vi "ReadFileONLY.vi"(8 "error in (no error)":errorcluster, 10 "file path (dialog if empty)":path) -> (0 "error out":errorcluster, 1 "Waveform Graph":waveform(dbl)[](graph), 2 "number of waveforms":i32, 3 "Array":string[](array[string]), 4 "saturated":bool[](array[boolean]), 5 "dX/dt 2":dbl[](graph))   [LabVIEW 2013]
uses:
  <instrlib>/niHWS/nihws.llb/niHWS Open File Permissions ID.ctl
  <instrlib>/niHWS/nihws.llb/niHWS Read Analog WDT.vi
panel:
  out "Array 2":dbl[](array[numeric]) format="%#_6p"
  in  "index (row)":i32
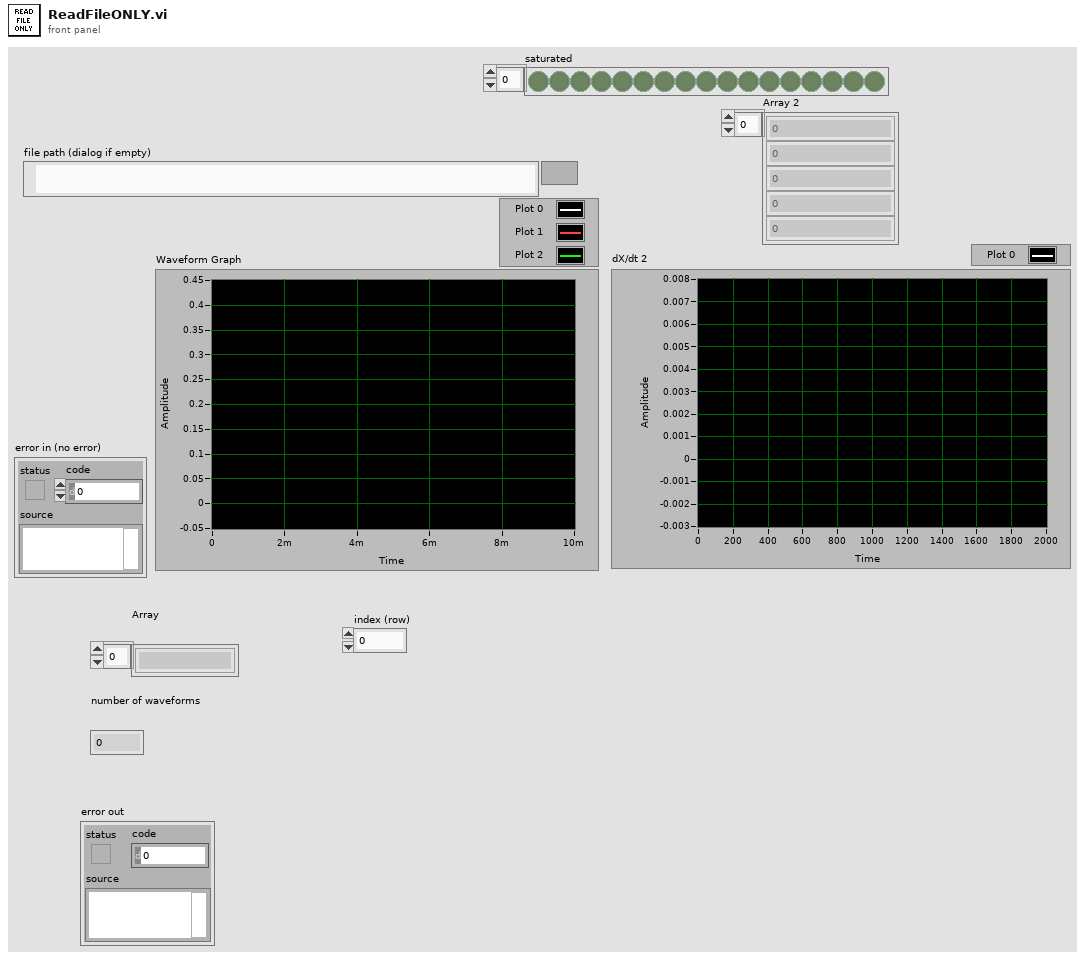
[diagram p1: front panel]
types:
  T1 = typedef "niHWS Open File Permissions ID.ctl" = enum32{"Read Only", "Read/Write Existing", "Read/Write/Create New", "Read/Write/Create New Always"}
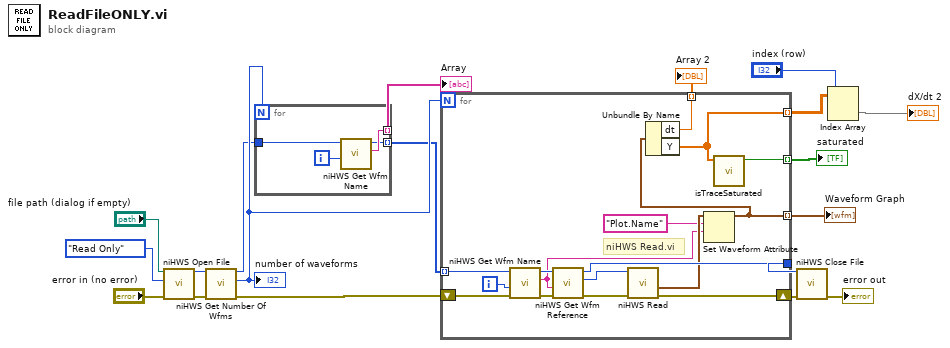
[diagram p0: block diagram]
diagram:
  n1 = call <instrlib>:"niHWS Open File.vi"("error in (no error)"="error in (no error)", "permissions (0:read only)"=niHWS_Open_File_Permissions_ID."Read Only", "file path"="file path (dialog if empty)") -> ("error out"=w10:errorcluster, "file handle"=w11:u32)  [unwired: 7 in]
  n2 = call <instrlib>:"niHWS Get Number Of Wfms.vi"("error in (no error)"=w10, "file handle in"=w11) -> ("error out"=w9:errorcluster, "number of waveforms"=w19:i32, "file handle out"=w16:u32)  [unwired: 7 in]
  "number of waveforms" <- w19
  n3 = for {
    N: w19 -> [_]
    tunnel: w16 -> [w23]
    tunnel: [w22] -> w18 mode=indexing
    tunnel: [w21] -> w17 mode=indexing
    i -> [w20]
    n4 = call <instrlib>:"niHWS Get Wfm Name.vi"("waveform index (0)"=w20, "file handle in"=w23) -> ("waveform name"=w22:string, "file handle out"=w21:u32)  [unwired: 7 in, 1 out]
  }
  "Array" <- w18
  n5 = for {
    N: w19 -> [_]
    tunnel: [w27] -> w6 mode=indexing
    tunnel: w17 -> [w38] mode=indexing
    tunnel: [w35] -> w15
    shift-right: [w37] -> w14
    shift-left: w9 -> [w39]
    tunnel: [w26] -> w5 mode=indexing
    tunnel: [w25] -> w4 mode=indexing
    tunnel: [w24] -> w1 mode=indexing
    i -> [w31]
    # "niHWS Read.vi"
    n6 = call <instrlib>:"niHWS Get Wfm Name.vi"("error in (no error)"=w39, "waveform index (0)"=w31, "file handle in"=w38) -> ("error out"=w33:errorcluster, "waveform name"=w29:string, "file handle out"=w36:u32)  [unwired: 6 in]
    n7 = call <instrlib>:"niHWS Get Wfm Reference.vi"("error in (no error)"=w33, "waveform name (empty)"=w29, "file handle in"=w36) -> ("error out"=w32:errorcluster, "waveform reference"=w34:u32, "file handle out"=w35:u32)  [unwired: 6 in]
    n8 = call-poly <instrlib>:"niHWS Read.vi"("error in (no error)"=w32, "waveform reference in"=w34) -> ("error out"=w37:errorcluster, "analog waveform"=w30:waveform(dbl))  [unwired: 6 in, 2 out]
    n9 = Set Waveform Attribute(5:w29, 6:"Plot.Name" ("name"), 7:w30) -> (3:w27:waveform(dbl))  [unwired: 1 in, 2 out]
    n10 = Unbundle By Name(w27) -> ("dt"=w24:dbl, "Y"=w26:dbl[])
    n11 = call "isTraceSaturated.vi"("dX/dt in"=w26) -> ("saturated"=w25:bool)  [unwired: 8 in, 2 out]
  }
  "Waveform Graph" <- w6
  "saturated" <- w4
  "Array 2" <- w1
  n12 = call <instrlib>:"niHWS Close File.vi"("error in (no error)"=w14, "file handle"=w15) -> ("error out"=→"error out":errorcluster)  [unwired: 9 in]
  n13 = Index Array(array=w5, index (row)="index (row)") -> (element=→"dX/dt 2":dbl[])  [unwired: 1 in]
